vi "test_libssh2_channel_signal_ex.vi"() -> ()   [LabVIEW 2013, in "libssh2_integration_tests.lvlib"]
uses:
  libssh2_integration_tests.lvlib
  <vilib>/addons/_JKI Toolkits/Caraya/classes/Test/Test.lvclass
  support/support.lvlib
  libssh2/libssh2.lvlib
  <vilib>/addons/_JKI Toolkits/Caraya/classes/Assert/Assert.lvclass
panel:
  out "error out":errorcluster
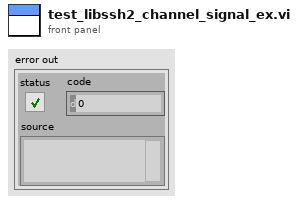
[diagram p1: front panel]
types:
  T1 = typedef "libssh2.lvlib/Session Refnum.ctl" = refnum<k1>
  T2 = typedef "libssh2.lvlib/Channel Refnum.ctl" = refnum<k1>
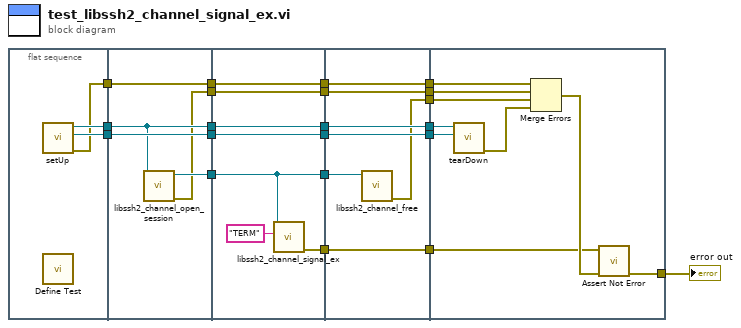
[diagram p0: block diagram]
diagram:
  n1 = flat-sequence {
    tunnel: [w24] -> w21
    tunnel: [w23] -> w20
    tunnel: [w22] -> w19
    tunnel: w21 -> [w28]
    tunnel: w20 -> [w29]
    tunnel: [w28] -> w5
    tunnel: [w29] -> w4
    tunnel: [w27] -> w3
    tunnel: w19 -> [w26]
    tunnel: [w26] -> w2
    tunnel: [w25] -> w1
    tunnel: w5 -> [w36]
    tunnel: [w36] -> w11
    tunnel: w4 -> [w35]
    tunnel: [w35] -> w10
    tunnel: w2 -> [w34]
    tunnel: [w34] -> w9
    tunnel: w1 -> [w33]
    tunnel: [w33] -> w8
    tunnel: w3 -> [w32]
    tunnel: [w32] -> w7
    tunnel: [w31] -> w6
    tunnel: w11 -> [w43]
    tunnel: w10 -> [w42]
    tunnel: [w43] -> w18
    tunnel: [w42] -> w17
    tunnel: [w41] -> w16
    tunnel: w9 -> [w40]
    tunnel: [w40] -> w15
    tunnel: w8 -> [w39]
    tunnel: [w39] -> w14
    tunnel: w7 -> [w38]
    tunnel: w6 -> [w37]
    tunnel: [w37] -> w12
    tunnel: w18 -> [w52]
    tunnel: w17 -> [w51]
    tunnel: [w50] -> w13
    tunnel: w16 -> [w48]
    tunnel: w15 -> [w47]
    tunnel: w14 -> [w45]
    tunnel: w12 -> [w44]
    frame #0 {
      n2 = call "setUp.vi"() -> ("error out"=w22:errorcluster, "connection ID"=w23:refnum<k5>, "session"=w24:T1)  [unwired: 9 in]
      n3 = call <vilib>:"Define Test.vi"() -> ()  [unwired: 10 in, 2 out]
    }
    frame #1 {
      n4 = call "libssh2_channel_open_session.vi"("session"=w28) -> ("error out"=w25:errorcluster, "channel"=w27:T2)  [unwired: 9 in]
    }
    frame #2 {
      n5 = call "libssh2_channel_signal_ex.vi"("signal name"="TERM", "channel"=w32) -> ("error out"=w31:errorcluster)  [unwired: 9 in]
    }
    frame #3 {
      n6 = call "libssh2_channel_free.vi"("channel"=w38) -> ("error out"=w41:errorcluster)  [unwired: 10 in]
    }
    frame #4 {
      n7 = call "tearDown.vi"("connection ID"=w51, "session"=w52) -> ("error out"=w49:errorcluster)  [unwired: 9 in]
      n8 = Merge Errors(w47, w45, w48, w49) -> (w46:errorcluster)
      n9 = call <vilib>:"Assert Not Error.vi"("error in (no error)"=w46, "Not Error?"=w44) -> ("error out"=w50:errorcluster)  [unwired: 8 in, 1 out]
    }
  }
  "error out" <- w13
